vi "Bring Up.vi"(8 "error in (no error)":errorcluster, 11 "Assembler in":refnum<class "Assembler.lvclass">) -> (0 "error out":errorcluster, 3 "Assembler out":refnum<class "Assembler.lvclass">)   [LabVIEW 2016, in "CLD Exam - ATM.lvlib" / "Assembler.lvclass"]
uses:
  Assembler.lvclass
  Assembler.lvclass/Assembler.ctl
  User Interface/User Interface.lvclass
  Terminal Timeout/Terminal Timeout.lvclass
  Terminal Menus/Terminal Menus.lvclass
  Terminal Message/Terminal Message.lvclass
  Bank Account/Bank Account.lvclass
  Replay/Replay.lvclass
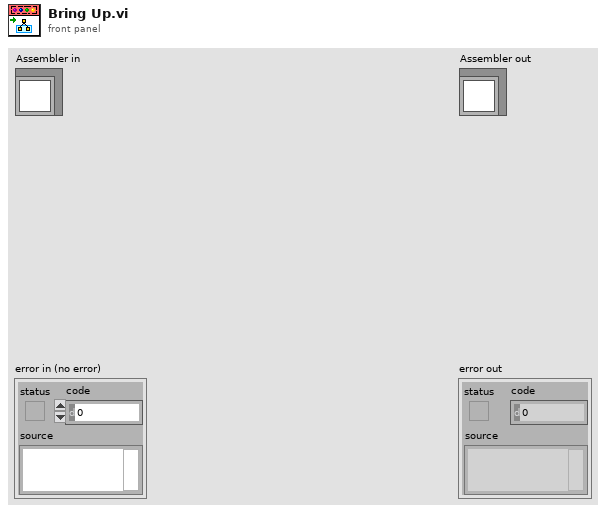
[diagram p1: front panel]
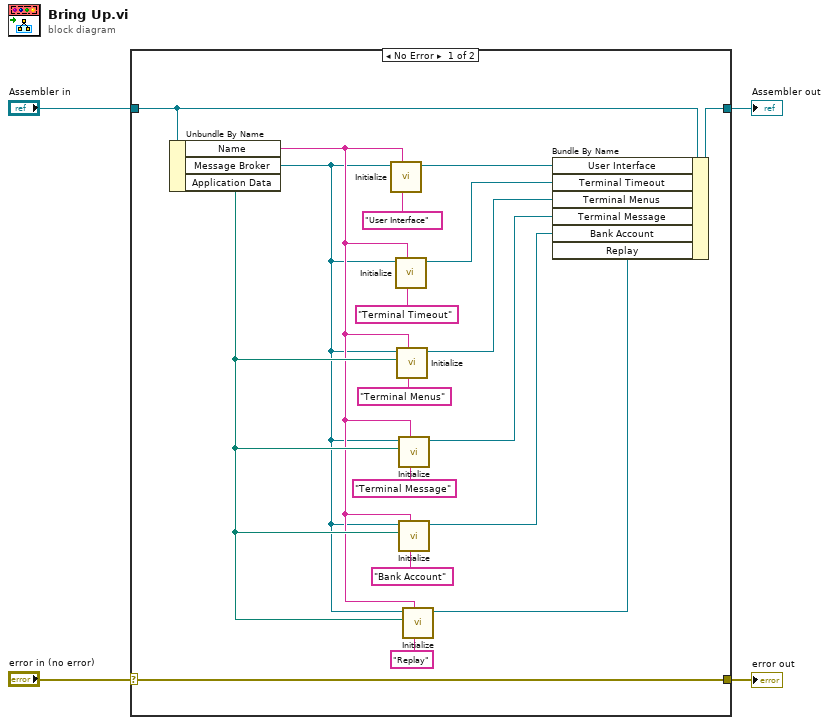
[diagram p0: block diagram]
diagram:
  n1 = case shown="No Error" "error in (no error)" {
    selector: "error in (no error)" -> [w22 w24]
    tunnel: [w22 w24] -> w3
    tunnel: [w18 w23] -> w1
    tunnel: "Assembler in" -> [w19 w23]
    frame No Error {
      n2 = Unbundle By Name(w19) -> ("Name"=w7:string, "Message Broker"=w5:refnum<class "Message Broker Interface Ref.lvclass">, "Application Data"=w8:path)
      n3 = call "Initialize.vi"("Actor Name"="User Interface", "Host Name"=w7, "Message Broker"=w5) -> ("User Interface out"=w20:refnum<class "User Interface.lvclass">)  [unwired: 7 in, 1 out]
      n4 = call "Initialize.vi"("Actor Name"="Terminal Timeout", "Host Name"=w7, "Message Broker"=w5) -> ("Terminal Timeout out"=w17:refnum<class "Terminal Timeout.lvclass">)  [unwired: 7 in, 1 out]
      n5 = call "Initialize.vi"("Actor Name"="Terminal Menus", "Host Name"=w7, "Application Data"=w8, "Message Broker"=w5) -> ("Terminal Menus out"=w14:refnum<class "Terminal Menus.lvclass">)  [unwired: 6 in, 1 out]
      n6 = call "Initialize.vi"("Actor Name"="Terminal Message", "Host Name"=w7, "Application Data"=w8, "Message Broker"=w5) -> ("Terminal Message out"=w13:refnum<class "Terminal Message.lvclass">)  [unwired: 6 in, 1 out]
      n7 = call "Initialize.vi"("Actor Name"="Bank Account", "Host Name"=w7, "Application Data"=w8, "Message Broker"=w5) -> ("Bank Account out"=w10:refnum<class "Bank Account.lvclass">)  [unwired: 6 in, 1 out]
      n8 = call "Initialize.vi"("Actor Name"="Replay", "Host Name"=w7, "Application Data"=w8, "Message Broker"=w5) -> ("Replay out"=w9:refnum<class "Replay.lvclass">)  [unwired: 6 in, 1 out]
      n9 = Bundle By Name(cluster=w19, "User Interface"=w20, "Terminal Timeout"=w17, "Terminal Menus"=w14, "Terminal Message"=w13, "Bank Account"=w10, "Replay"=w9) -> (w18:refnum<class "Assembler.lvclass">)
    }
    frame Error {
    }
  }
  "error out" <- w3
  "Assembler out" <- w1
